vi "Check project version.vi"(11 "path to XML document":path) -> ()   [LabVIEW 2015]
uses:
  <vilib>/xml/Load XML File.vi
  <vilib>/xml/Close Reference(Node).vi
  <resource>/objmgr/DOMUserDefRef.rc
  <vilib>/xml/NI_XML.lvlib
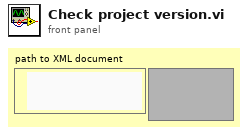
[diagram p1: front panel]
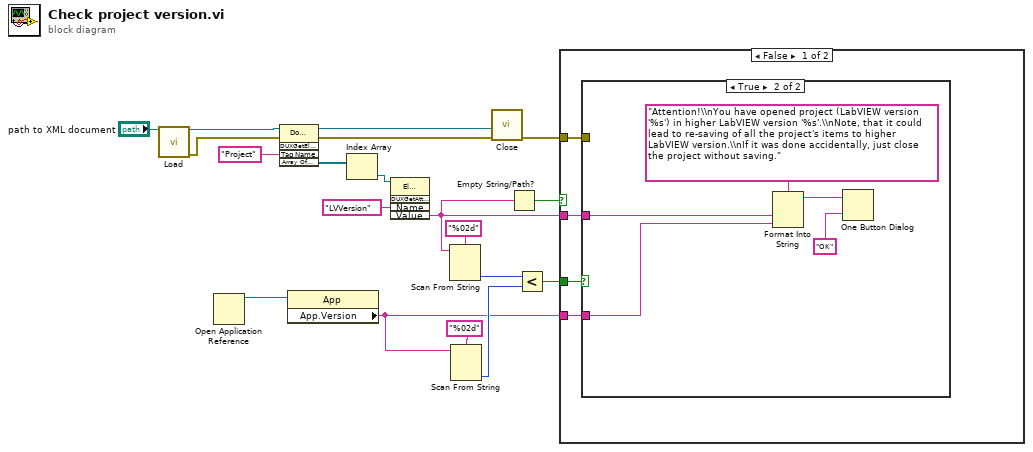
[diagram p0: block diagram]
diagram:
  n1 = call-poly <vilib>:"Load.vi"("path to XML document"="path to XML document") -> ("DOM document out"=w18:refnum<k20>, "error out"=w16:errorcluster)  [unwired: 12 in, 1 out]
  n2 = Open Application Reference() -> (3:w9:refnum<vi>)  [unwired: 4 in, 1 out]
  n3 = invoke class="Document" method="DUXGetElementsByTagName"(reference=w18, error in=w16, "Tag Name"="Project") -> (reference out=w14:refnum<k20>, error out=w15:errorcluster, "Array Of Elements"=w13:refnum<k20>[])  [unwired: 2 in, 2 out]
  n4 = property on="Property Node" class="App"(reference=w9) -> ("App.Version"=w3:string)  [unwired: 1 in, 2 out]
  n5 = Index Array(array=w13) -> (element=w12:refnum<k20>)  [unwired: 1 in]
  n6 = invoke on="Invoke Node" class="Element" method="DUXGetAttribute"(reference=w12, "Name"="LVVersion") -> ("Value"=w2:string)  [unwired: 3 in, 4 out]
  n7 = Scan From String(format string="%02d", input string=w2) -> (output 1=w7:i32)  [unwired: 3 in, 3 out]
  n8 = Scan From String(format string="%02d", input string=w3) -> (output 1=w6:i32)  [unwired: 3 in, 3 out]
  n9 = call-poly <vilib>:"Close.vi"("error in (no error)"=w15, "node"=w14) -> ("error out"=w4:errorcluster)  [unwired: 7 in]
  n10 = Empty String/Path?(string/path=w2) -> (empty?=w1:bool)
  n11 = Less?(x=w7, y=w6) -> (x < y?=w5:bool)
  n12 = case shown="False" w1 {
    tunnel: w5 -> [w23 _]
    tunnel: w4 -> [w22 _]
    tunnel: w3 -> [w21 _]
    tunnel: w2 -> [w20 _]
    frame False {
      n13 = case shown="True" w23 {
        tunnel: w22 -> [_ _]
        tunnel: w20 -> [_ w25]
        tunnel: w21 -> [_ w24]
        frame False {
        }
        frame True {
          n14 = Format Into String(format string="Attention!\\nYou have opened project (LabVIEW version '%s') in higher LabVIEW version '%s'.\\nNote, that it could lead to re-saving of all the project's items to higher LabVIEW version.\\nIf it was done accidentally, just close the project without saving.", w25, w24) -> (resulting string=w27:string)  [unwired: 2 in, 1 out]
          n15 = One Button Dialog(message=w27, button name ("OK")="OK") -> ()  [unwired: 1 out]
        }
      }
    }
    frame True {
    }
  }
